vi "Get Data Offset (x0).vi"(11 "data attributes":variant) -> (1 "x0":dbl format="%_8g", 3 "data attributes":variant)   [LabVIEW 2017]
uses:
  <vilib>/addons/_NISVFA/_Shared subVIs/Controls/NI Channel Properties.ctl
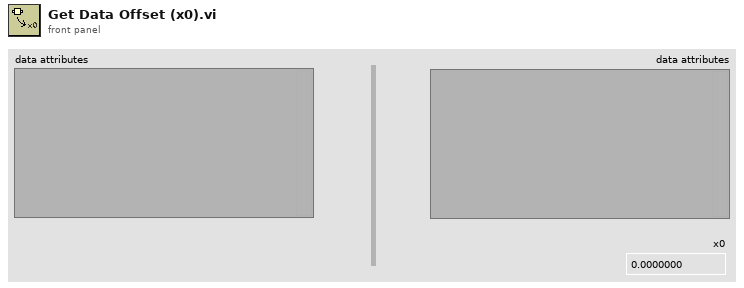
[diagram p1: front panel]
types:
  T1 = typedef "NI Channel Properties.ctl" = u16
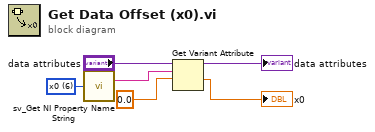
[diagram p0: block diagram]
diagram:
  w6 = T1 6 items=["Channel name", "Channel description", "Y-axis label", "Y-axis unit string", "X-axis label", "X-axis unit string", "x0", "dx", "Number of samples", "X channel", "Filter settled", "dB reference", "Window", "Window parameter", "Window size", "FFT size", "Peak units", "Spectrum type", "Magnitude scale", "Spectral density"] ("property")
  n1 = call <vilib>:"sv_Get NI Property Name String.vi"("property"=w6) -> ("TDMS property name"=w5:string)  [unwired: 13 in, 1 out]
  n2 = Get Variant Attribute(Variant="data attributes", name=w5, default value (empty Variant)=0.0) -> (duplicate Variant=→"data attributes":variant, value=→"x0":dbl)  [unwired: 1 in, 2 out]
